vi "popUPSINO.vi"() -> (3 "estadoConsulta":bool=TRUE)   [LabVIEW 2014]
panel:
  in  "ControlNo":bool caption="Presione No para Rechazar"
  in  "ControlSi":bool caption="Presione Si para Aceptar"
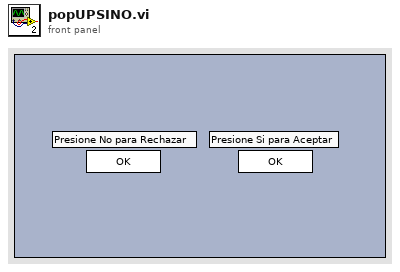
[diagram p1: front panel]
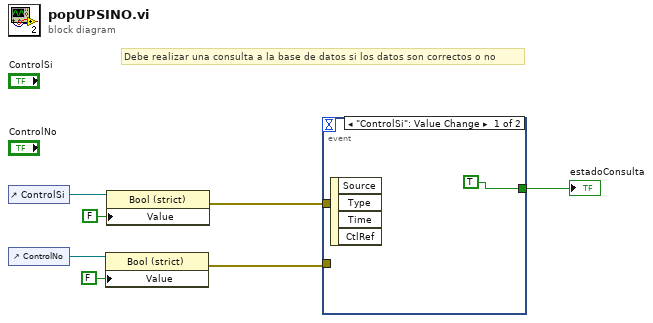
[diagram p0: block diagram]
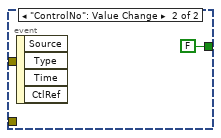
[diagram p2: hidden frame]
diagram:
  # "Debe realizar una consulta a la base de datos si los datos son correctos o no"
  n1 = control-ref of="ControlSi"() -> (w6:refnum<vi>)
  n2 = control-ref of="ControlNo"() -> (w4:refnum<vi>)
  n3 = property class="Bool (strict)"(reference=w4, "Value"=FALSE) -> (error out=w1:errorcluster)  [unwired: 1 in, 1 out]
  n4 = property class="Bool (strict)"(reference=w6, "Value"=FALSE) -> (error out=w2:errorcluster)  [unwired: 1 in, 1 out]
  n5 = event shown="[0] \"ControlSi\": Value Change" {
    selector: _ -> [_ _]
    dyn-events: _ -> [_ _]
    timeout: _ -> [_ _]
    tunnel: [TRUE ("estadoConsulta") FALSE ("estadoConsulta")] -> w7
    tunnel: w2 -> [_ _]
    tunnel: w1 -> [_ _]
    event "ControlSi": Value Change {
      n6 = event-data() -> ()  [unwired: 1 in, 4 out]
    }
    event "ControlNo": Value Change {
      n7 = event-data() -> ()  [unwired: 1 in, 4 out]
    }
  }
  "estadoConsulta" <- w7
